vi "Destroy.vi"(8 "Error in":errorcluster, 10 "Unhandled Msgs":refnum<class "Msg.lvclass">[](array[class]), 11 "TEMPLATE Actor in":refnum<class "TEMPLATE Actor.lvclass">) -> (3 "TEMPLATE Actor out":refnum<class "TEMPLATE Actor.lvclass">)   [LabVIEW 2025, in "TEMPLATE Actor.lvlib" / "TEMPLATE Actor.lvclass"]
uses:
  TEMPLATE Actor.lvclass
  <vilib>/Nathan Davis/jettl/jettl/jettl/Msg/Msg.lvclass
  TEMPLATE Actor.lvclass/TEMPLATE Actor.ctl
  <vilib>/Nathan Davis/jettl/jettl/jettl/Actor/Actor/Actor.lvclass
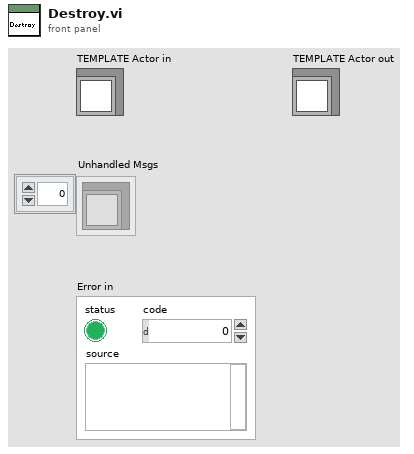
[diagram p1: front panel]
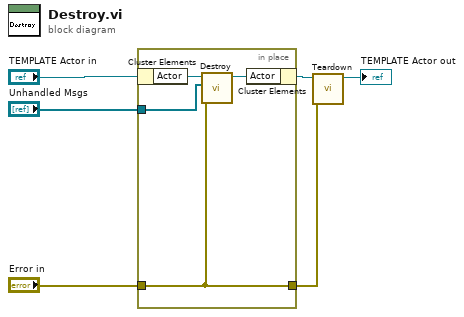
[diagram p0: block diagram]
diagram:
  n1 = in-place {
    in-place-border: "Error in" -> [w7]
    in-place-border: "Unhandled Msgs" -> [w8]
    in-place-border: [w7] -> w1
    n2 = in-place-cluster #1("TEMPLATE Actor in") -> ("Actor"=w10:refnum<class "Actor.lvclass">)
    n3 = call-dynamic "Destroy.vi"("Error in"=w7, "Unhandled Msgs"=w8, "Actor in"=w10) -> ("Actor out"=w9:refnum<class "Actor.lvclass">)  [unwired: 8 in]
    n4 = in-place-cluster #1("Actor"=w9) -> (w3:refnum<class "TEMPLATE Actor.lvclass">)
  }
  n5 = call "Teardown.vi"("Error in"=w1, "TEMPLATE Actor in"=w3) -> ("TEMPLATE Actor out"=→"TEMPLATE Actor out":refnum<class "TEMPLATE Actor.lvclass">)  [unwired: 9 in]
